vi "AO N Samples FPGA（Host）.vi"() -> ()   [LabVIEW 2019]
uses:
  <vilib>/FPGAPlugInAG/ELVIS III/niLvFpga_Open_ELVIS III.vi
  <vilib>/rvi/interface/common/dynamic/niFpgaDynamicAddResources.vi
  <vilib>/rvi/interface/common/niFpgaWaitOnOcc.vi
  <vilib>/Utility/error.llb/Error Cluster From Error Code.vi
  <vilib>/rvi/errors/niLvFpgaAdjustHostInterfaceError.vi
  <vilib>/FPGAPlugInAG/Dynamic/niLvFpga_Run_Dynamic.vi
  <vilib>/FPGAPlugInAG/Dynamic/niLvFpga_Abort_Dynamic.vi
  <vilib>/FPGAPlugInAG/Dynamic/niLvFpga_Close_Dynamic.vi
  <vilib>/rvi/interface/nirviOpenFPGA/nirviOpenFPGA.xnode
  FPGA Bitfiles/aiofpga_FPGATarget_AONSamplesFPGA_vUIBqh-I+ug.lvbitx
  AO N Samples FPGA.vi
  <vilib>/rvi/interface/nirviMethod/nirviMethod.xnode
  <vilib>/rvi/interface/nirviReadWriteControl/nirviReadWriteControl.xnode
  <vilib>/rvi/interface/nirviCloseFPGA/nirviCloseFPGA.xnode
  <vilib>/FPGAPlugInAG/Dynamic/niLvFpga_ConfigureFifo_Dynamic.vi
  <vilib>/rvi/errors/niLvFpgaMergeErrorWithErrorCode.vi
  NiFpgaLv.dll
  <vilib>/rvi/interface/Simulation/niFpgaSimulationCallBeginRW.vi
  <vilib>/FPGAPlugInAG/Dynamic/niLvFpga_WriteFifo_Dynamic.vi
panel:
  in  "采样点数":u32=1000
  in  "B1 信号频率":dbl=400.0
  in  "B0 信号频率":dbl=200.0
  in  "A1 信号频率":dbl=100.0
  in  "A0 信号频率":dbl=10.0
  in  "最大采样点数":dbl=10000.0
  in  "采样率 [Hz]":dbl=10000.0 min=1000.0 max=1600000.0
  out "B1":dbl[](graph)
  out "B0":dbl[](graph)
  out "A1":dbl[](graph)
  out "A0":dbl[](graph)
  in  "停止":bool
  in  "Enable":bool[](array[boolean])=[TRUE, FALSE, FALSE, FALSE]
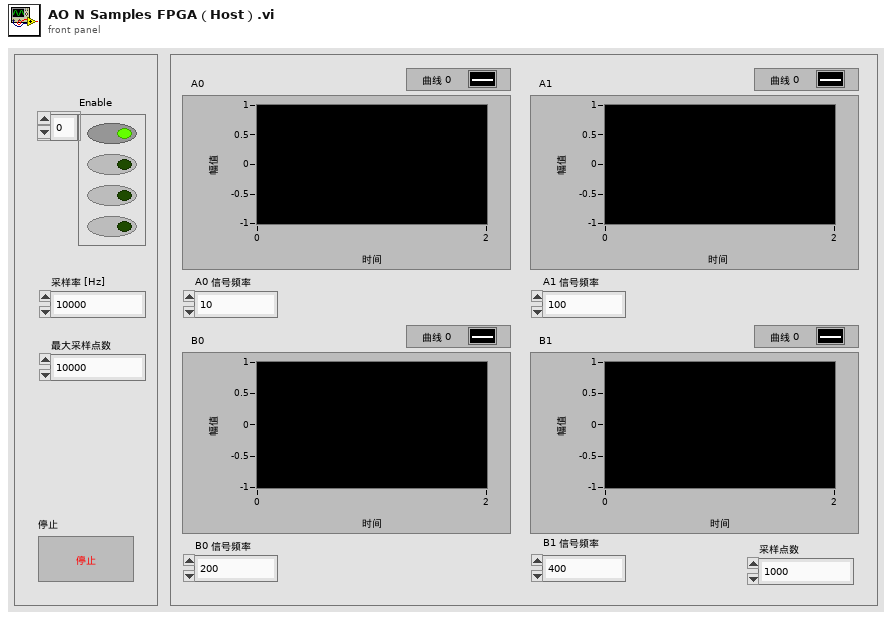
[diagram p1: front panel]
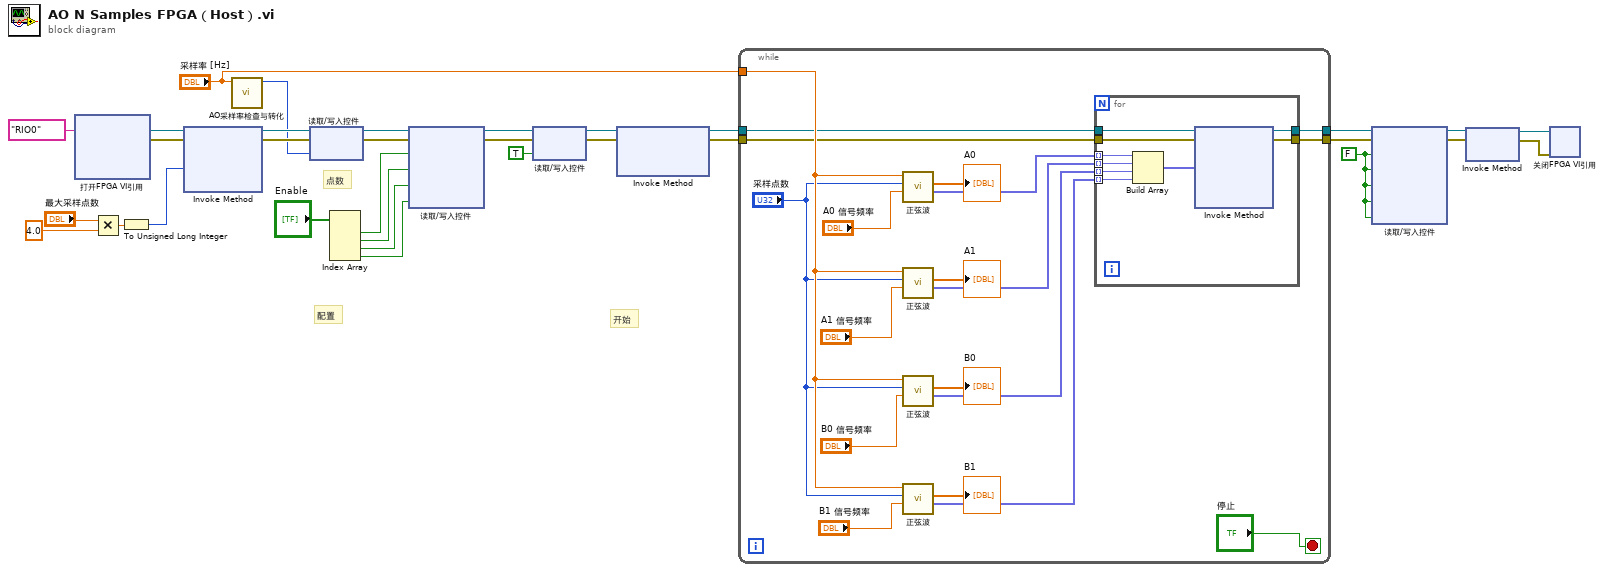
[diagram p0: block diagram]
diagram:
  w5 = FALSE ("开始")
  # "开始"
  # "配置"
  # "点数"
  n1 = xnode "打开FPGA VI引用"("资源名称"=tag "RIO0") -> ("FPGA VI引用输出"=w31:refnum<k20>, "错误输出"=w30:errorcluster)  [unwired: 1 in]
  n2 = Multiply(x="最大采样点数", y=4.0) -> (x*y=w27:dbl)
  n3 = To Unsigned Long Integer(number=w27) -> (unsigned 32bit integer=w26:u32)
  n4 = xnode "Invoke Method"("FPGA VI引用输入"=w31, "错误输入"=w30, "请求的深度"=w26) -> ("FPGA VI引用输出"=w10:refnum<k20>, "错误输出"=w13:errorcluster)  [unwired: 1 out]
  n5 = call "AO采样率检查与转化.vi"("AO FIFO Sample Rate"="采样率 [Hz]") -> ("Count (tick/s)"=w9:u32)  [unwired: 9 in, 1 out]
  n6 = xnode "读取/写入控件"("FPGA VI引用输入"=w10, "错误输入"=w13, "CNTR"=w9) -> ("FPGA VI引用输出"=w11:refnum<k20>, "错误输出"=w12:errorcluster)
  n7 = Index Array(array="Enable") -> (element #1=w21:bool, element #2=w22:bool, element #3=w23:bool, element #4=w24:bool)  [unwired: 4 in]
  n8 = xnode "读取/写入控件"("FPGA VI引用输入"=w11, "错误输入"=w12, "A0.Enable"=w21, "A1.Enable"=w22, "B0.Enable"=w23, "B1.Enable"=w24) -> ("FPGA VI引用输出"=w19:refnum<k20>, "错误输出"=w20:errorcluster)
  n9 = xnode "读取/写入控件"("FPGA VI引用输入"=w19, "错误输入"=w20, "开始"=TRUE) -> ("FPGA VI引用输出"=w16:refnum<k20>, "错误输出"=w17:errorcluster)
  n10 = xnode "Invoke Method"("FPGA VI引用输入"=w16, "错误输入"=w17) -> ("FPGA VI引用输出"=w14:refnum<k20>, "错误输出"=w15:errorcluster)  [unwired: 1 in]
  n11 = while {
    tunnel: w15 -> [w36]
    tunnel: w14 -> [w37]
    tunnel: "采样率 [Hz]" -> [w51]
    tunnel: [w35] -> w7
    tunnel: [w34] -> w6
    stop <- "停止" stop-if-true
    n12 = call "正弦波.vi"("信号频率 Hz"="A0 信号频率", "采样点数 S"="采样点数", "采样率 [Hz]"=w51) -> ("Sine 波形 FXP"=w41:fxp<+/-,20,5>[], "Sine 波形"=→"A0":dbl[])  [unwired: 7 in]
    n13 = call "正弦波.vi"("信号频率 Hz"="A1 信号频率", "采样点数 S"="采样点数", "采样率 [Hz]"=w51) -> ("Sine 波形 FXP"=w40:fxp<+/-,20,5>[], "Sine 波形"=→"A1":dbl[])  [unwired: 7 in]
    n14 = call "正弦波.vi"("信号频率 Hz"="B0 信号频率", "采样点数 S"="采样点数", "采样率 [Hz]"=w51) -> ("Sine 波形 FXP"=w39:fxp<+/-,20,5>[], "Sine 波形"=→"B0":dbl[])  [unwired: 7 in]
    n15 = call "正弦波.vi"("信号频率 Hz"="B1 信号频率", "采样点数 S"="采样点数", "采样率 [Hz]"=w51) -> ("Sine 波形 FXP"=w38:fxp<+/-,20,5>[], "Sine 波形"=→"B1":dbl[])  [unwired: 7 in]
    n16 = for {
      tunnel: w41 -> [w60] mode=indexing
      tunnel: w40 -> [w59] mode=indexing
      tunnel: w39 -> [w58] mode=indexing
      tunnel: w38 -> [w57] mode=indexing
      tunnel: w37 -> [w56]
      tunnel: w36 -> [w55]
      tunnel: [w53] -> w35
      tunnel: [w52] -> w34
      n17 = Build Array(w60, w59, w58, w57) -> (w54:fxp<+/-,20,5>[])
      n18 = xnode "Invoke Method"("FPGA VI引用输入"=w56, "错误输入"=w55, "数据"=w54) -> ("FPGA VI引用输出"=w52:refnum<k20>, "错误输出"=w53:errorcluster)  [unwired: 1 in, 1 out]
    }
  }
  n19 = xnode "读取/写入控件"("FPGA VI引用输入"=w6, "错误输入"=w7, "开始"=w5, "A0.Enable"=w5, "A1.Enable"=w5, "B0.Enable"=w5, "B1.Enable"=w5) -> ("FPGA VI引用输出"=w3:refnum<k20>, "错误输出"=w4:errorcluster)
  n20 = xnode "Invoke Method"("FPGA VI引用输入"=w3, "错误输入"=w4) -> ("FPGA VI引用输出"=w1:refnum<k20>, "错误输出"=w2:errorcluster)
  n21 = xnode "关闭FPGA VI引用"("FPGA VI引用输入"=w1, "错误输入"=w2) -> ()  [unwired: 1 out]
